vi "DSF Configuration to cluster.vi"(8 "error in (no error)":errorcluster, 11 "DSFConfiguration in":refnum<class "DSFConfiguration.lvclass">) -> (0 "error out":errorcluster, 3 "configuration cluster":T1)   [LabVIEW 2017, in "DSFConfiguration.lvclass"]
uses:
  DSFConfiguration.lvclass
  Controls/dsf configuration.ctl
  Controls/dsf plugin.ctl
  Controls/dsf timing.ctl
  Controls/dsf group.ctl
  Controls/dsf transfer.ctl
  Controls/dsf channel.ctl
  Controls/dsf settings.ctl
  DSFConfiguration.lvclass/DSFConfiguration.ctl
  IDable/IDable.lvclass/IDable.ctl
  DSFPlugin/DSFPlugin.lvclass/DSFPlugin.ctl
  DSFPluginSettings/DSFPluginSettings.lvclass/DSFPluginSettings.ctl
  DSFChannel/DSFChannel.lvclass/DSFChannel.ctl
  DSFGroup/DSFGroup.lvclass/DSFGroup.ctl
  DSFTransfer/DSFTransfer.lvclass/DSFTransfer.ctl
  DSFPluginSettings/DSFPluginSettings.lvclass
  C:/github/data-sharing-framework/Source/Configuration API/Classes/IDable/IDable.lvclass
  DSFChannel/DSFChannel.lvclass
  DSFGroup/DSFGroup.lvclass
  DSFPlugin/DSFPlugin.lvclass
  DSFTransfer/DSFTransfer.lvclass
  IDable/IDable.lvclass
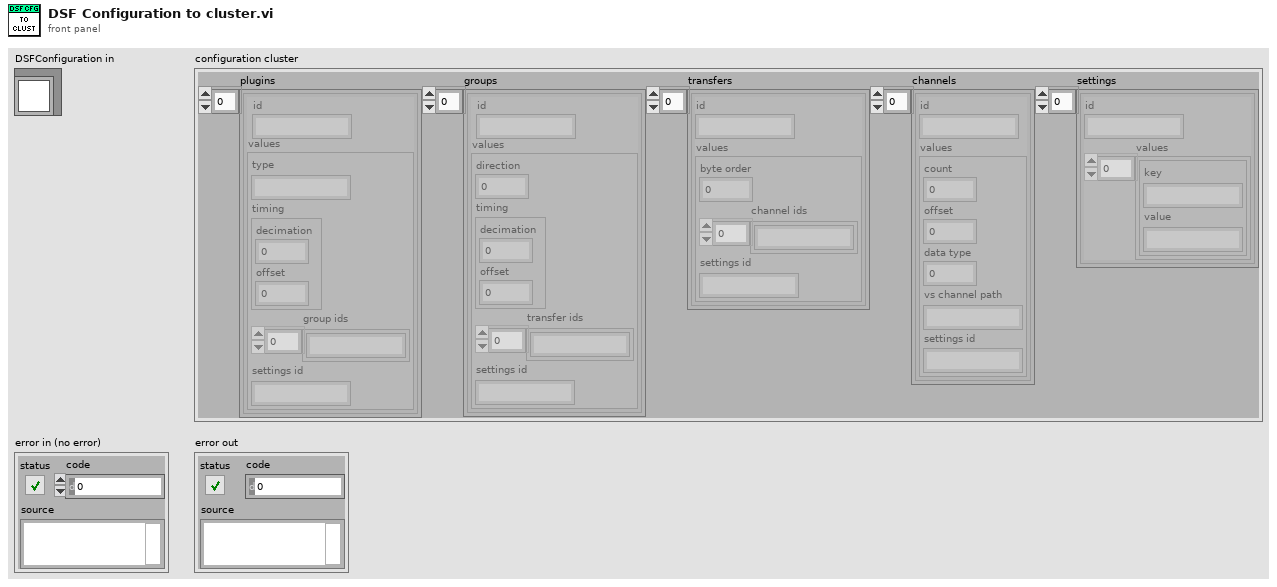
[diagram p1: front panel]
types:
  T1 = typedef "dsf configuration.ctl" = cluster{"plugins":cluster{"id":string, "values":T2}[], "groups":cluster{"id":string, "values":T4}[], "transfers":cluster{"id":string, "values":T5}[], "channels":cluster{"id":string, "values":T6}[], "settings":cluster{"id":string, "values":T7}[]}
  T2 = typedef "dsf plugin.ctl" = cluster{"type":string, "timing":T3, "group ids":string[], "settings id":string}
  T3 = typedef "dsf timing.ctl" = cluster{"decimation":i32, "offset":i32}
  T4 = typedef "dsf group.ctl" = cluster{"direction":i32, "timing":T3, "transfer ids":string[], "settings id":string}
  T5 = typedef "dsf transfer.ctl" = cluster{"byte order":i32, "channel ids":string[], "settings id":string}
  T6 = typedef "dsf channel.ctl" = cluster{"count":i32, "offset":i32, "data type":i32, "vs channel path":string, "settings id":string}
  T7 = typedef "dsf settings.ctl" = cluster{"key":string, "value":string}[]
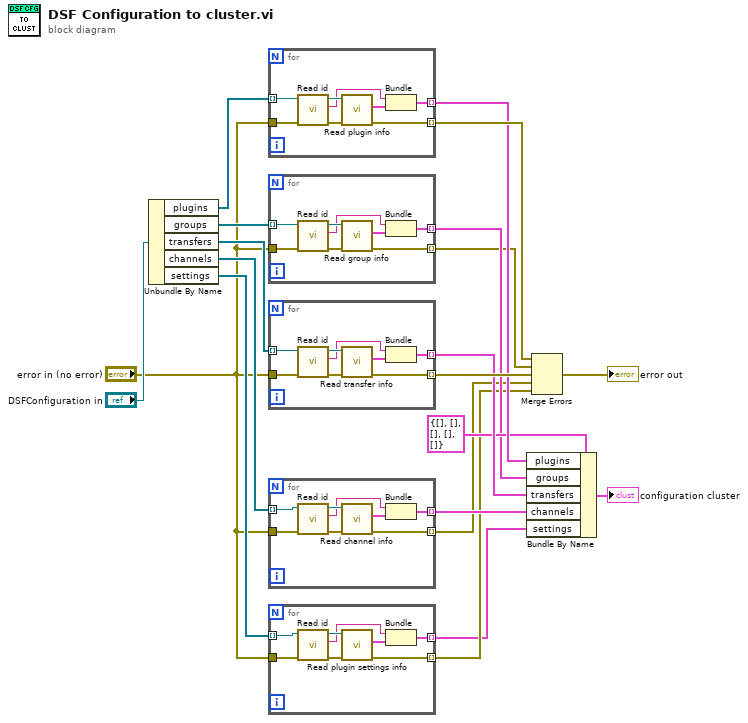
[diagram p0: block diagram]
diagram:
  n1 = Unbundle By Name("DSFConfiguration in") -> ("plugins"=w12:refnum<class "DSFPlugin.lvclass">[], "groups"=w10:refnum<class "DSFGroup.lvclass">[], "transfers"=w11:refnum<class "DSFTransfer.lvclass">[], "channels"=w7:refnum<class "DSFChannel.lvclass">[], "settings"=w4:refnum<class "DSFPluginSettings.lvclass">[])
  n2 = for {
    tunnel: w12 -> [w27] mode=indexing
    tunnel: [w28] -> w17 mode=indexing
    tunnel: "error in (no error)" -> [w25]
    tunnel: [w24] -> w18 mode=indexing
    n3 = call "Read id.vi"("error in (no error)"=w25, "IDable in"=w27) -> ("error out"=w22:errorcluster, "id"=w23:string, "IDable out"=w26:refnum<class "DSFPlugin.lvclass">)  [unwired: 7 in]
    n4 = call "Read plugin info.vi"("error in (no error)"=w22, "DSFPlugin in"=w26) -> ("error out"=w24:errorcluster, "plugin info"=w21:T2)  [unwired: 7 in, 1 out]
    n5 = Bundle("id"=w23, "plugin info"=w21) -> (w28:cluster{"id":string, "plugin info":T2})  [unwired: 1 in]
  }
  n6 = for {
    tunnel: w10 -> [w35] mode=indexing
    tunnel: [w36] -> w9 mode=indexing
    tunnel: "error in (no error)" -> [w33]
    tunnel: [w32] -> w8 mode=indexing
    n7 = call "Read id.vi"("error in (no error)"=w33, "IDable in"=w35) -> ("error out"=w30:errorcluster, "id"=w31:string, "IDable out"=w34:refnum<class "DSFGroup.lvclass">)  [unwired: 7 in]
    n8 = call "Read group info.vi"("error in (no error)"=w30, "DSFGroup in"=w34) -> ("error out"=w32:errorcluster, "group info"=w29:T4)  [unwired: 7 in, 1 out]
    n9 = Bundle("id"=w31, "group info"=w29) -> (w36:cluster{"id":string, "group info":T4})  [unwired: 1 in]
  }
  n10 = for {
    tunnel: w11 -> [w42] mode=indexing
    tunnel: [w44] -> w16 mode=indexing
    tunnel: "error in (no error)" -> [w41]
    tunnel: [w37] -> w19 mode=indexing
    n11 = call "Read id.vi"("error in (no error)"=w41, "IDable in"=w42) -> ("error out"=w38:errorcluster, "id"=w40:string, "IDable out"=w43:refnum<class "DSFTransfer.lvclass">)  [unwired: 7 in]
    n12 = call "Read transfer info.vi"("error in (no error)"=w38, "DSFTransfer in"=w43) -> ("error out"=w37:errorcluster, "transfer info"=w39:T5)  [unwired: 7 in, 1 out]
    n13 = Bundle("id"=w40, "transfer info"=w39) -> (w44:cluster{"id":string, "transfer info":T5})  [unwired: 1 in]
  }
  n14 = for {
    tunnel: w7 -> [w51] mode=indexing
    tunnel: [w52] -> w6 mode=indexing
    tunnel: "error in (no error)" -> [w49]
    tunnel: [w48] -> w5 mode=indexing
    n15 = call "Read id.vi"("error in (no error)"=w49, "IDable in"=w51) -> ("error out"=w46:errorcluster, "id"=w47:string, "IDable out"=w50:refnum<class "DSFChannel.lvclass">)  [unwired: 7 in]
    n16 = call "Read channel info.vi"("error in (no error)"=w46, "DSFChannel in"=w50) -> ("error out"=w48:errorcluster, "channel info"=w45:T6)  [unwired: 7 in, 1 out]
    n17 = Bundle("id"=w47, "channel info"=w45) -> (w52:cluster{"id":string, "channel info":T6})  [unwired: 1 in]
  }
  n18 = for {
    tunnel: w4 -> [w59] mode=indexing
    tunnel: [w60] -> w1 mode=indexing
    tunnel: "error in (no error)" -> [w57]
    tunnel: [w56] -> w2 mode=indexing
    n19 = call "Read id.vi"("error in (no error)"=w57, "IDable in"=w59) -> ("error out"=w54:errorcluster, "id"=w55:string, "IDable out"=w58:refnum<class "DSFPluginSettings.lvclass">)  [unwired: 7 in]
    n20 = call "Read plugin settings info.vi"("error in (no error)"=w54, "DSFPluginSettings in"=w58) -> ("error out"=w56:errorcluster, "plugin settings info"=w53:T7)  [unwired: 7 in, 1 out]
    n21 = Bundle("id"=w55, "plugin settings info"=w53) -> (w60:cluster{"id":string, "plugin settings info":T7})  [unwired: 1 in]
  }
  n22 = Bundle By Name(cluster=T1 {"plugins"=[], "groups"=[], "transfers"=[], "channels"=[], "settings"=[]}, "plugins"=w17, "groups"=w9, "transfers"=w16, "channels"=w6, "settings"=w1) -> (→"configuration cluster":T1)
  n23 = Merge Errors(w18, w8, w19, w5, w2) -> (→"error out":errorcluster)
